vi "Flatten and Save Class Data.vi"(8 "error in":errorcluster, 11 "Loopback in":refnum<class "Loopback.lvclass">) -> (0 "error out":errorcluster, 3 "Loopback out":refnum<class "Loopback.lvclass">)   [LabVIEW 2020, in "Loopback.lvclass"]
uses:
  Loopback.lvclass
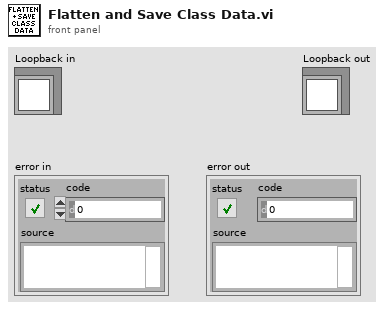
[diagram p1: front panel]
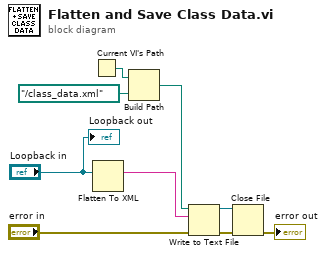
[diagram p0: block diagram]
diagram:
  n1 = Current VI's Path() -> (path=w5:path)
  n2 = Flatten To XML(6:"Loopback in") -> (2:w8:string)
  n3 = Build Path(base path=w5, name or relative path=path "../class_data.xml") -> (appended path=w7:path)
  n4 = Write to Text File(file (use dialog)=w7, text=w8, error in="error in") -> (refnum out=w1:refnum<file>, error out=w9:errorcluster)  [unwired: 1 in, 1 out]
  n5 = Close File(refnum=w1, error in=w9) -> (error out=→"error out":errorcluster)  [unwired: 1 out]
  "Loopback out" <- "Loopback in"
